vi "kpro 2016.vi"(0 "Output KPRO":path=path "c:/junk.dat", 1 "Initialize":bool, 2 "Finished In":bool, 5 "Absolute Depth In":sgl format="%.2f", 7 "Total Volume In":dbl format="%.2f", 9 "Zeroed Pressure":dbl format="%.2f", 11 "Flow":dbl format="%.2f", 12 "Read String Pot":bool, 13 "Increment":bool, 14 "SS In":i32) -> (4 "Finished Out":bool, 6 "SS Out":i32, 8 "Current Depth Out":sgl format="%.2f", 10 "Total Volume Out":dbl format="%.2f", 15 "Output Array":dbl[][](array[numeric])=[[17182499.0, -1.0, -1.0, 0.07295542423579193, 10.0, 30.0, 1.0, 0.2942041776993234, 33.989999999999995], [17194122.0, -2.0, -2.0, 0.08603630732168976, 10.0, 30.0, 1.0, 0.28579594169762795, 34.989999999999995], [17196835.0, -3.0, -3.0, 0.36859565057132326, 10.0, 30.0, 1.0, 0.27785495971103086, 35.989999999999995], [17198861.0, -4.0, -4.0, 0.493583415597236, 10.0, 30.0, 1.0, 0.27034333603676675, 36.989999999999995], [17203069.0, -5.0, -5.0, 0.23764258555133078, 10.0, 30.0, 1.0, 0.2632271650434325, 37.989999999999995], [17204351.0, -6.0, -6.0, 0.7800312012480499, 10.0, 30.0, 1.0, 0.2564760194921775, 38.989999999999995], [17205734.0, -7.0, -7.0, 0.7230657989877078, 10.0, 30.0, 1.0, 0.25006251562890724, 39.989999999999995], [17206879.0, -8.0, -8.0, 0.8733624454148472, 10.0, 30.0, 1.0, 0.24396194193705784, 40.989999999999995], [17208211.0, -9.0, -9.0, 0.7507507507507507, 10.0, 30.0, 1.0, 0.23815194093831868, 41.989999999999995], [17211804.0, -10.0, -10.0, 0.27831895352073477, 10.0, 30.0, 1.0, 0.23261223540358225, 42.989999999999995], [17214313.0, -11.0, -11.0, 0.3985651654045437, 10.0, 30.0, 1.0, 0.22732439190725168, 43.989999999999995], [17215593.0, -12.0, -12.0, 0.78125, 10.0, 30.0, 1.0, 0.22227161591464772, 44.989999999999995], [17216822.0, -13.0, -13.0, 0.8136696501220504, 10.0, 30.0, 1.0, 0.21743857360295718, 45.989999999999995], [17218103.0, -14.0, -14.0, 0.7806401249024201, 10.0, 30.0, 1.0, 0.2128112364332837, 46.989999999999995], [17219267.0, -15.0, -15.0, 0.859106529209622, 10.0, 30.0, 1.0, 0.20837674515524068, 47.989999999999995], [17220448.0, -16.0, -16.0, 0.8467400508044031, 10.0, 30.0, 1.0, 0.20412329046744235, 48.989999999999995], [17221627.0, -17.0, -17.0, 0.8481764206955046, 10.0, 30.0, 1.0, 0.20004000800160035, 49.989999999999995], [17222775.0, -18.0, -18.0, 0.8710801393728224, 10.0, 30.0, 1.0, 0.19611688566385568, 50.989999999999995], [17223888.0, -19.0, -19.0, 0.8984725965858041, 10.0, 30.0, 1.0, 0.19234468166955185, 51.989999999999995], [17225019.0, -20.0, -20.0, 0.8841732979664014, 10.0, 30.0, 1.0, 0.18871485185884132, 52.989999999999995], [17226151.0, -21.0, -21.0, 0.88339222614841, 10.0, 30.0, 1.0, 0.18521948508983146, 53.989999999999995], [17227282.0, -22.0, -22.0, 0.8841732979664014, 10.0, 30.0, 1.0, 0.18185124568103292, 54.989999999999995]] format="%.5f")   [LabVIEW 2016]
uses:
  Waterloo DAQ/controls/Kpro hydraulic measurement cluster.ctl
  Waterloo DAQ/controls/MCC DAQ Readings.ctl
  KPRO_lv2015/Kpro Globals.vi
  <vilib>/Utility/file.llb/Write Delimited Spreadsheet (DBL).vi
panel:
  in  "String Pot \nSlope":dbl=1.7339999675750732 format="%.2f"
  in  "Sensor Cluster In":T1
  in  "Cluster":T2
  out "Current Absolute Depth":dbl
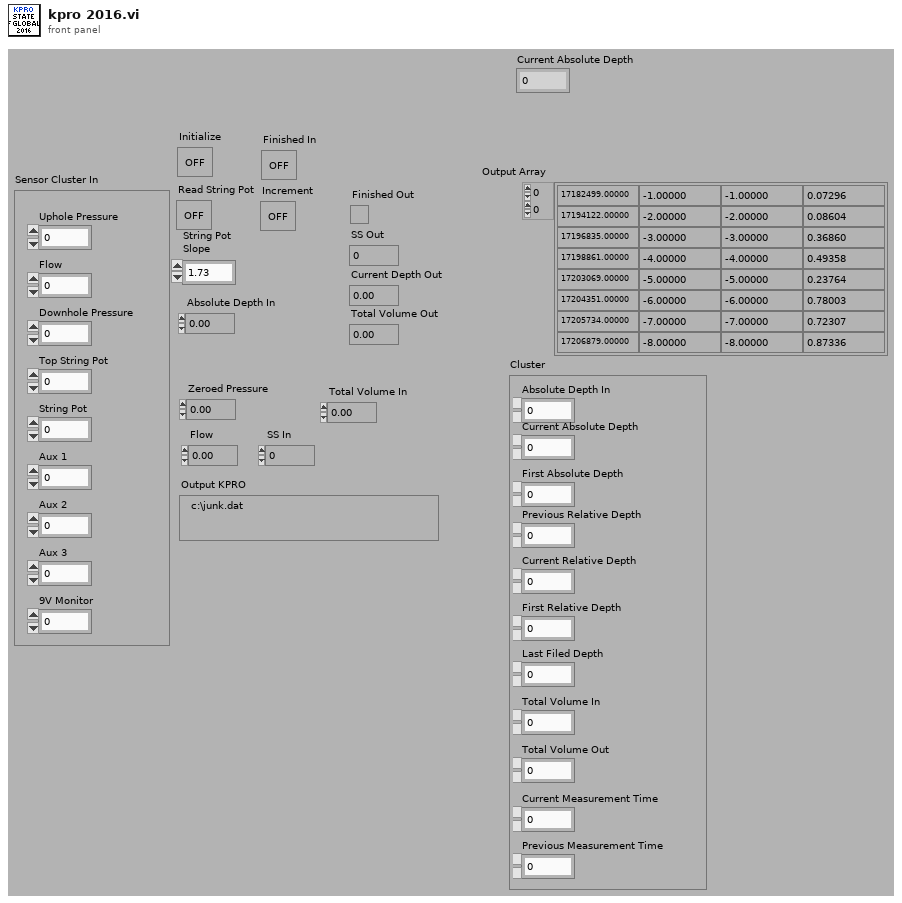
[diagram p1: front panel]
types:
  T1 = typedef "MCC DAQ Readings.ctl" = cluster{"Uphole Pressure":dbl, "Flow":dbl, "Downhole Pressure":dbl, "Top String Pot":dbl, "String Pot":dbl, "Aux 1":dbl, "Aux 2":dbl, "Aux 3":dbl, "9V Monitor":dbl}
  T2 = typedef "Kpro hydraulic measurement cluster.ctl" = cluster{"Absolute Depth In":dbl, "Current Absolute Depth":dbl, "First Absolute Depth":dbl, "Previous Relative Depth":dbl, "Current Relative Depth":dbl, "First Relative Depth":dbl, "Last Filed Depth":dbl, "Total Volume In":dbl, "Total Volume Out":dbl, "Current Measurement Time":dbl, "Previous Measurement Time":dbl}
  T3 = enum16{"Initialize", "Read", "Calc IK and generate Array", "Write Data & finish"}
  T4 = enum16{"Initialize", "Read", "read2", "Write Data & finish"}
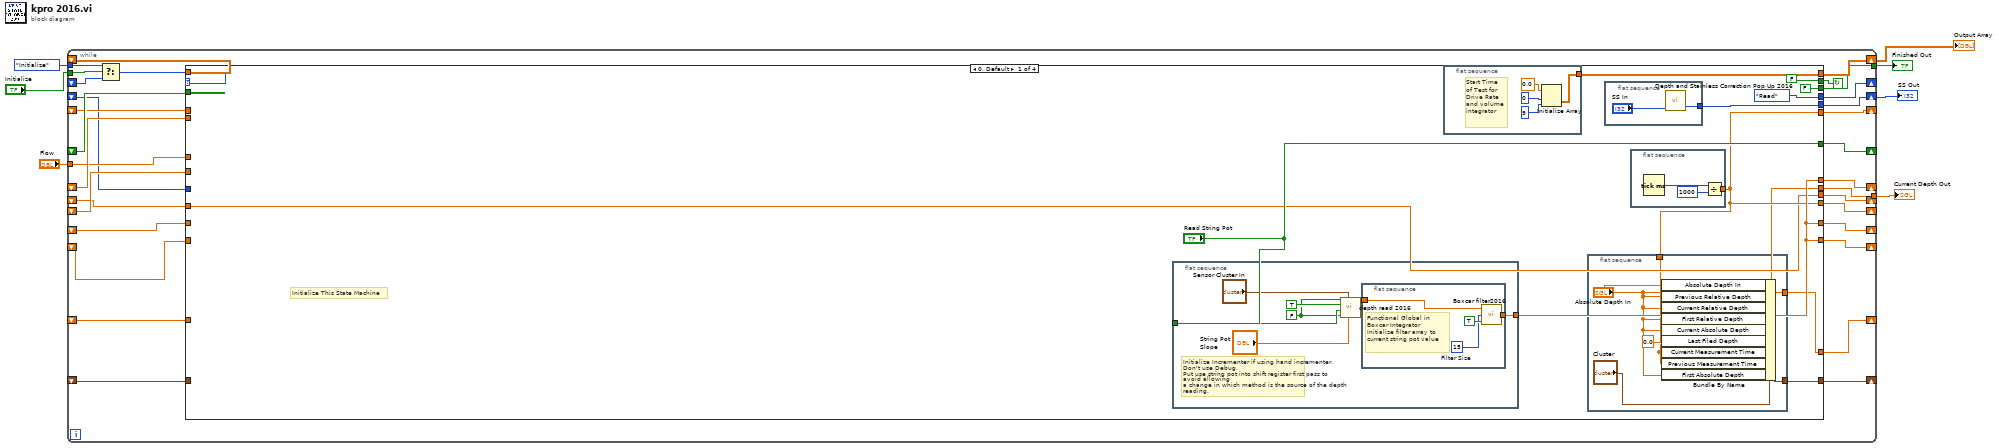
[diagram p0: block diagram]
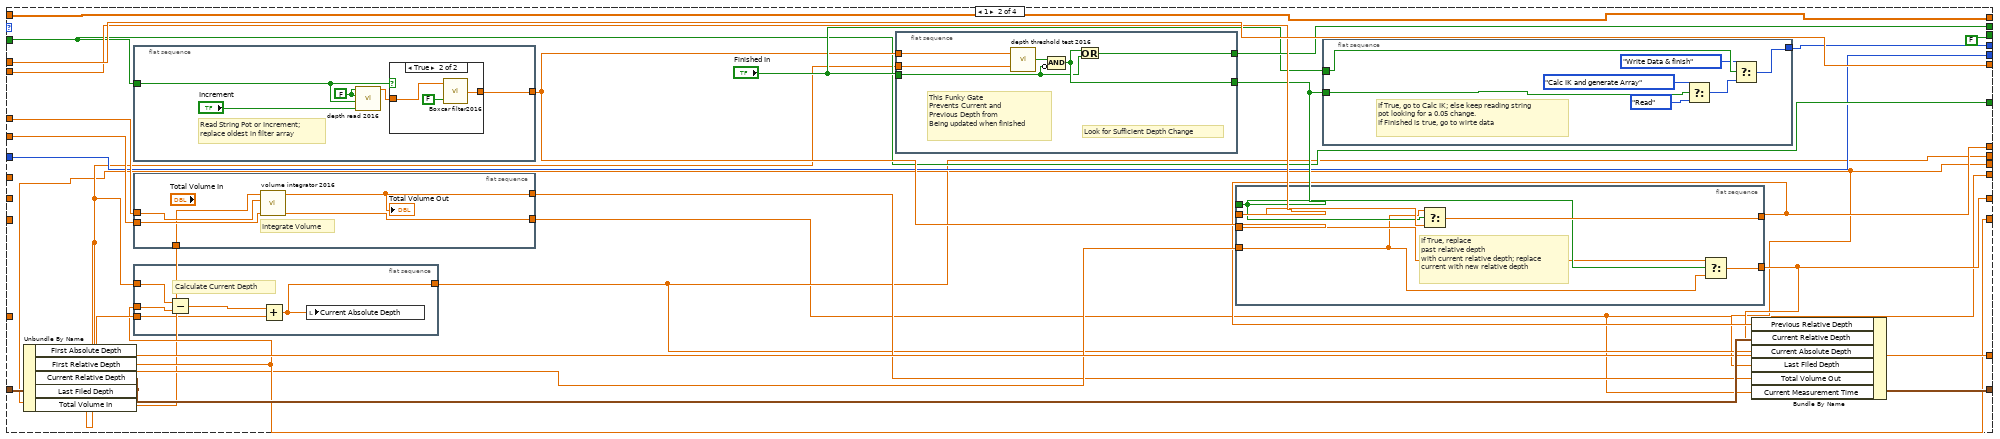
[diagram p2: hidden frame]
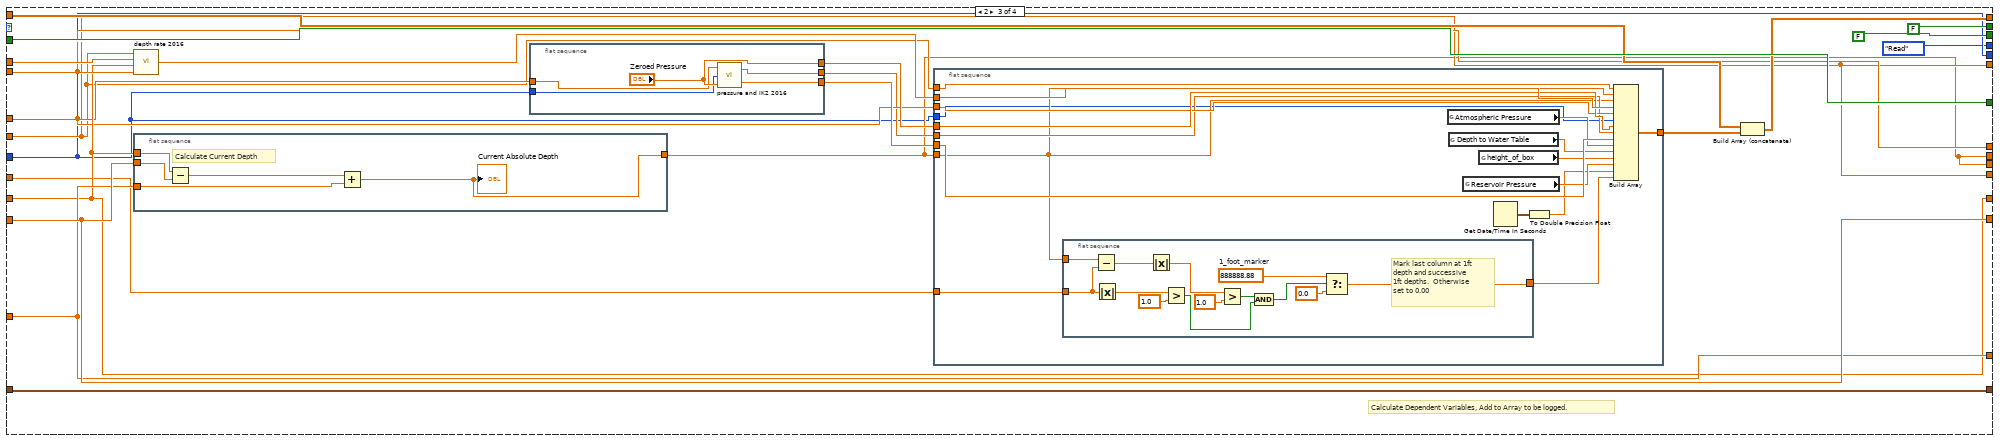
[diagram p4: hidden frame]
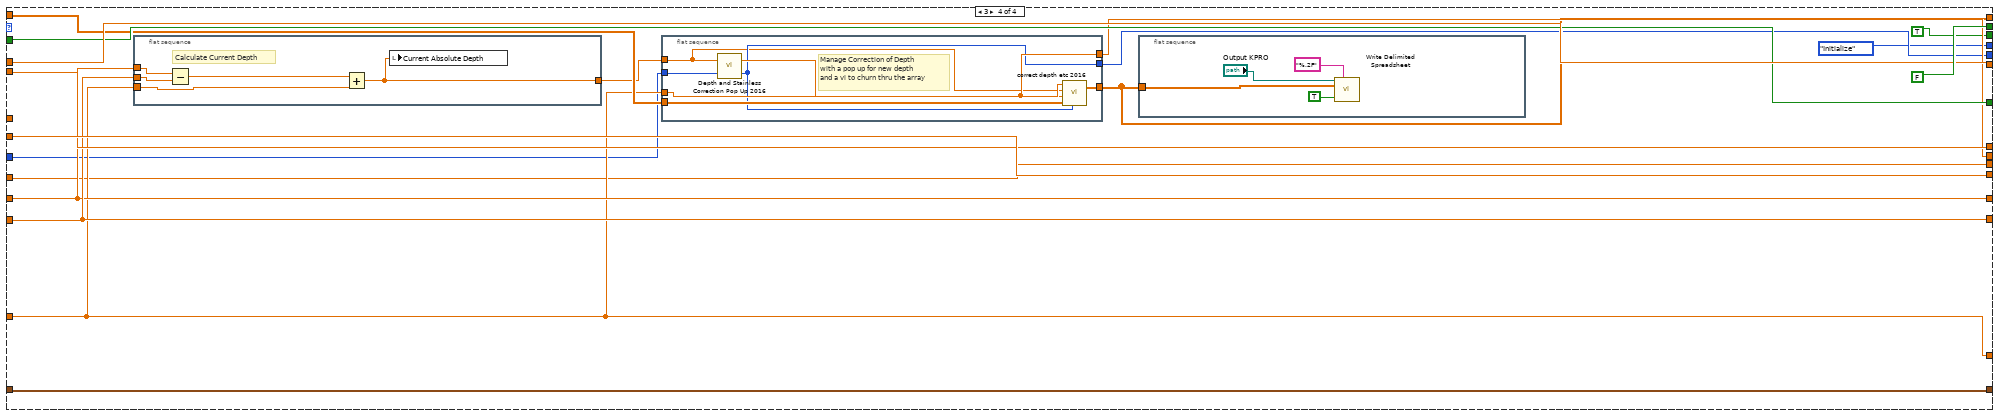
[diagram p5: hidden frame]
diagram:
  n1 = while {
    shift-left: _ -> [w15]
    shift-right: [w16] -> _
    shift-left: _ -> [w18]
    shift-right: [w17] -> w2
    tunnel: [w19] -> w3
    tunnel: [w20] -> w4
    shift-left: _ -> [w21]
    shift-right: [w22] -> _
    shift-left: _ -> [w23]
    shift-right: [w24] -> w1
    shift-left: _ -> [w25]
    shift-right: [w26] -> _
    tunnel: "Flow" -> [w28]
    shift-left: _ -> [w30]
    shift-right: [w31] -> _
    shift-left: _ -> [w29]
    shift-right: [w32] -> _
    shift-left: _ -> [w27]
    shift-right: [w33] -> _
    shift-left: _ -> [w34]
    shift-right: [w35] -> _
    shift-left: _ -> [w36]
    shift-right: [w37] -> _
    tunnel: "Initialize" -> [w38]
    tunnel: T3."Initialize" -> [w13]
    shift-left: _ -> [w11]
    shift-right: [w10] -> _
    shift-right: [w9] -> _
    shift-left: _ -> [w8]
    stop <- w14 continue-if-true
    n2 = Select(t=w13, s=w38, f=w11) -> (s? t:f=w12:u16)
    n3 = case shown="0, Default" w12 {
      tunnel: [T4."Read" w97 T3."Read" T3."Initialize"] -> w10
      tunnel: [w48 w83 w151 w212] -> w37
      tunnel: w36 -> [_ _ w151 w212]
      tunnel: ["Read String Pot" w88 w159 w214] -> w35
      tunnel: w34 -> [_ w88 w159 w214]
      tunnel: [w41 w98 w143 w215] -> w33
      tunnel: [w41 w75 w143 w216] -> w32
      tunnel: [w48 w79 w153 w213] -> w31
      tunnel: w30 -> [_ w94 w153 w213]
      tunnel: w29 -> [_ w96 w143 w216]
      tunnel: w28 -> [_ w95 w145 _]
      tunnel: w27 -> [_ w98 w154 w215]
      tunnel: [w48 w78 w147 w211] -> w26
      tunnel: w25 -> [_ _ w147 w211]
      tunnel: [w47 w99 w156 w207] -> w24
      tunnel: w23 -> [_ w99 w157 w210]
      tunnel: [w39 w84 w150 w208] -> w22
      tunnel: w21 -> [_ _ w150 w208]
      tunnel: [w39 w77 w142 w209] -> w20
      tunnel: [FALSE w93 FALSE FALSE] -> w14
      tunnel: [FALSE FALSE FALSE TRUE] -> w19
      tunnel: w18 -> [_ w87 w140 w205]
      tunnel: [w44 w87 w140 w204] -> w17
      tunnel: [w40 w76 w142 w203] -> w16
      tunnel: w15 -> [w40 _ w141 w203]
      tunnel: [w42 w86 w138 w200] -> w9
      tunnel: w8 -> [_ w85 w138 w200]
      frame 0, Default {
        # "Initialize This State Machine"
        n4 = flat-sequence {
          tunnel: "Read String Pot" -> [w64]
          tunnel: [w62] -> w48
          frame #0 {
            w63 = FALSE
            # "Initialize Incrementer if using hand incrementer,\nDon't use Debug,\nPut use string pot into shift register first pass to avoid allowing\na change in which method is the source of the depth reading."
            n5 = call "depth read 2016.vi"("String Pot \nSlope"="String Pot \nSlope", "Sensor Cluster In"="Sensor Cluster In", "Increment Button"=w63, "Read String Pot"=w64, "Initialize Debug"=TRUE, "Debug"=w63) -> ("Distance"=w66:dbl)  [unwired: 5 in]
            n6 = flat-sequence {
              tunnel: w66 -> [w68]
              tunnel: [w67] -> w62
              frame #0 {
                w69 = 15  # Filter Size
                # "Functional Global in \nBoxcar Integrator\nInitialize filter array to \ncurrent string pot value"
                n7 = call "Boxcar filter2016.vi"("Initialize"=TRUE, "Filter Size"=w69, "Filter Input"=w68) -> ("Filter Output"=w67:dbl)
              }
            }
          }
        }
        n8 = flat-sequence {
          tunnel: [w74] -> w47
          frame #0 {
            # "Start Time\nof Test for\nDrive Rate\nand volume\nintegrator"
            n9 = Initialize Array(0.0, 0, 9) -> (w74:dbl[][])
          }
        }
        n10 = flat-sequence {
          tunnel: [w56] -> w42
          tunnel: w41 -> [w54]
          tunnel: ["Absolute Depth In"] -> w39
          frame #0 {
            n11 = Bundle By Name(cluster="Cluster", "Absolute Depth In"="Absolute Depth In", "Previous Relative Depth"="Absolute Depth In", "Current Relative Depth"="Absolute Depth In", "First Relative Depth"="Absolute Depth In", "Current Absolute Depth"="Absolute Depth In", "Last Filed Depth"=0.0, "Current Measurement Time"=w54, "Previous Measurement Time"=w54, "First Absolute Depth"="Absolute Depth In") -> (w56:T2)
          }
        }
        n12 = flat-sequence {
          tunnel: [w50] -> w44
          frame #0 {
            n13 = call "Depth and Stainless Correction Pop Up 2016.vi"("New Number\n of Stainless\n(Count)"="SS In") -> ("Feet of\nStainless to be\nUsed (Count)"=w50:i32)  [unwired: 1 in, 1 out]
          }
        }
        n14 = flat-sequence {
          tunnel: [w57] -> w41
          frame #0 {
            n15 = Tick Count (ms)() -> (millisecond timer value=w59:u32)
            n16 = Divide(x=w59, y=u32 1000) -> (x/y=w57:dbl)
          }
        }
      }
      frame 1 {
        n17 = Unbundle By Name(w85) -> ("First Absolute Depth"=w84:dbl, "First Relative Depth"=w83:dbl, "Current Relative Depth"=w82:dbl, "Last Filed Depth"=w76:dbl, "Total Volume In"=w81:dbl)
        n18 = flat-sequence {
          tunnel: [w112] -> w89
          tunnel: w88 -> [w111]
          frame #0 {
            w114 = FALSE
            # "Read String Pot or Increment;\nreplace oldest in filter array"
            n19 = call "depth read 2016.vi"("Increment Button"="Increment", "Read String Pot"=w111, "Initialize Debug"=w114, "Debug"=w114) -> ("Distance"=w115:dbl)  [unwired: 7 in]
            n20 = case shown="True" w111 {
              tunnel: w115 -> [w116 w118]
              tunnel: [w116 w117] -> w112
              frame False {
              }
              frame True {
                n21 = call "Boxcar filter2016.vi"("Initialize"=FALSE, "Filter Input"=w118) -> ("Filter Output"=w117:dbl)  [unwired: 1 in]
              }
            }
          }
        }
        n22 = flat-sequence {
          tunnel: w96 -> [w110]
          tunnel: [w109] -> w75
          tunnel: w95 -> [w108]
          tunnel: w81 -> [w107]
          tunnel: [w106] -> w80
          frame #0 {
            # "Integrate Volume"
            n23 = call "volume integrator 2016.vi"("Previous Time (sec)"=w110, "Flow"=w108, "Total Volume in"=w107) -> ("Current Time (sec)"=w109:dbl, "Total Volume Out"=w106:dbl)  [unwired: 3 in]
            "Total Volume Out" <- w106
          }
        }
        n24 = flat-sequence {
          tunnel: w83 -> [w137]
          tunnel: w84 -> [w135]
          tunnel: w82 -> [w134]
          tunnel: [w133] -> w77
          frame #0 {
            # "Calculate Current Depth"
            n25 = Subtract(x=w134, y=w137) -> (x-y=w136:dbl)
            n26 = Add(x=w136, y=w135) -> (x+y=w133:dbl)
            n27 = local write "Current Absolute Depth"(w133) -> ()
          }
        }
        n28 = flat-sequence {
          tunnel: [w124] -> w93
          tunnel: [w123] -> w92
          tunnel: "Finished In" -> [w122]
          tunnel: w89 -> [w121]
          tunnel: w82 -> [w120]
          frame #0 {
            # "Look for Sufficient Depth Change"
            # "This Funky Gate\nPrevents Current and \nPrevious Depth from \nBeing updated when finished"
            n29 = call "depth threshold test 2016.vi"("Depth\nPrevious"=w120, "Depth \nCurrent"=w121) -> ("Threshold\nExceeded"=w125:bool)
            n30 = Compound Arithmetic op=AND(w125, invert w122) -> (w123:bool)
            n31 = Or(x=w123, y=w122) -> (x .or. y?=w124:bool)
          }
        }
        n32 = flat-sequence {
          tunnel: [w105] -> w79
          tunnel: w94 -> [w104]
          tunnel: [w103] -> w78
          tunnel: w92 -> [w102]
          tunnel: w89 -> [w101]
          tunnel: w82 -> [w100]
          frame #0 {
            # "If True, replace\npast relative depth\nwith current relative depth; replace\ncurrent with new relative depth"
            n33 = Select(t=w100, s=w102, f=w104) -> (s? t:f=w105:dbl)
            n34 = Select(t=w101, s=w102, f=w100) -> (s? t:f=w103:dbl)
          }
        }
        n35 = flat-sequence {
          tunnel: [w132] -> w97
          tunnel: w92 -> [w130]
          tunnel: "Finished In" -> [w129]
          frame #0 {
            # "If True, go to Calc IK; else keep reading string pot looking for a 0.05 change.\nIf Finished is true, go to wirte data"
            n36 = Select(t=T3."Calc IK and generate Array", s=w130, f=T3."Read") -> (s? t:f=w131:T3)
            n37 = Select(t=T3."Write Data & finish", s=w129, f=w131) -> (s? t:f=w132:T3)
          }
        }
        n38 = Bundle By Name(cluster=w85, "Previous Relative Depth"=w79, "Current Relative Depth"=w78, "Current Absolute Depth"=w77, "Last Filed Depth"=w76, "Total Volume Out"=w80, "Current Measurement Time"=w75) -> (w86:T2)
      }
      frame 2 {
        # "Calculate Dependent Variables, Add to Array to be logged."
        n39 = call "depth rate 2016.vi"("Depth Last"=w153, "Depth Current"=w147, "Time Last"=w154, "Time Current"=w143) -> ("Depth Rate"=w152:dbl)
        n40 = flat-sequence {
          tunnel: w151 -> [w198]
          tunnel: w150 -> [w197]
          tunnel: w147 -> [w196]
          tunnel: [w195] -> w142
          frame #0 {
            # "Calculate Current Depth"
            n41 = Subtract(x=w196, y=w198) -> (x-y=w199:dbl)
            n42 = Add(x=w199, y=w197) -> (x+y=w195:dbl)
            "Current Absolute Depth" <- w195
          }
        }
        n43 = flat-sequence {
          tunnel: [w194] -> w158
          tunnel: ["Zeroed Pressure"] -> w149
          tunnel: w145 -> [w192]
          tunnel: [w191] -> w144
          tunnel: w140 -> [w190]
          frame #0 {
            n44 = call "pressure and IK2 2016.vi"("Pressure"="Zeroed Pressure", "Ft. of SS"=w190, "flow"=w192) -> ("Corrected Headloss"=w194:dbl, "IK"=w191:dbl)
          }
        }
        n45 = flat-sequence {
          tunnel: w158 -> [w176]
          tunnel: [w175] -> w155
          tunnel: w152 -> [w174]
          tunnel: w149 -> [w173]
          tunnel: w145 -> [w172]
          tunnel: w144 -> [w171]
          tunnel: w143 -> [w166]
          tunnel: w142 -> [w164]
          tunnel: w141 -> [w162]
          tunnel: w140 -> [w160]
          frame #0 {
            n46 = flat-sequence {
              tunnel: w164 -> [w189]
              tunnel: [w183] -> w163
              tunnel: w162 -> [w179]
              frame #0 {
                w185 = 888888.88  # 1_foot_marker
                # "Mark last column at 1ft \ndepth and successive\n1ft depths.  Otherwise\nset to 0.00"
                n47 = Subtract(x=w189, y=w179) -> (x-y=w188:dbl)
                n48 = Absolute Value(x=w179) -> (abs(x)=w177:dbl)
                n49 = Absolute Value(x=w188) -> (abs(x)=w186:dbl)
                n50 = Greater?(x=w177, y=1.0) -> (0:w180:bool)
                n51 = Greater?(x=w186, y=1.0) -> (0:w181:bool)
                n52 = And(x=w181, y=w180) -> (x .and. y?=w182:bool)
                n53 = Select(t=w185, s=w182, f=0.0) -> (s? t:f=w183:dbl)
              }
            }
            n54 = global read "Kpro Globals.vi" "Atmospheric Pressure"() -> (w170:dbl)
            n55 = global read "Kpro Globals.vi" "Depth to Water Table"() -> (w168:dbl)
            n56 = global read "Kpro Globals.vi" "Reservoir Pressure"() -> (w169:dbl)
            n57 = global read "Kpro Globals.vi" "height_of_box"() -> (w167:dbl)
            n58 = Get Date/Time In Seconds() -> (seconds since 1Jan1904=w161:timestamp)
            n59 = To Double Precision Float(number=w161) -> (double precision float=w165:dbl)
            n60 = Build Array(w166, w164, w164, w174, w172, w160, w173, w171, w176, w170, w168, w167, w169, w165, w163) -> (w175:dbl[])
          }
        }
        n61 = Build Array (concatenate)(w157, w155) -> (w156:dbl[][])
      }
      frame 3 {
        n62 = flat-sequence {
          tunnel: w212 -> [w228]
          tunnel: w211 -> [w227]
          tunnel: w208 -> [w226]
          tunnel: [w225] -> w202
          frame #0 {
            # "Calculate Current Depth"
            n63 = Subtract(x=w227, y=w228) -> (x-y=w229:dbl)
            n64 = Add(x=w229, y=w226) -> (x+y=w225:dbl)
            n65 = local write "Current Absolute Depth"(w225) -> ()
          }
        }
        n66 = flat-sequence {
          tunnel: w210 -> [w224]
          tunnel: [w223] -> w209
          tunnel: w208 -> [w222]
          tunnel: [w221] -> w207
          tunnel: w205 -> [w220]
          tunnel: [w219] -> w204
          tunnel: w202 -> [w218]
          frame #0 {
            # "Manage Correction of Depth\nwith a pop up for new depth\nand a vi to churn thru the array"
            n67 = call "Depth and Stainless Correction Pop Up 2016.vi"("New Number\n of Stainless\n(Count)"=w220, "Input \nCorrected \nDepth (Feet)"=w218) -> ("Feet of\nStainless to be\nUsed (Count)"=w219:i32, "Depth to \nbe Used \n(Feet)"=w223:sgl)
            n68 = call "correct depth etc 2016.vi"("Correct Depth"=w223, "Incorrect Depth"=w218, "First Absolute Depth"=w222, "Uncorrected Array"=w224, "New Stainless Feet"=w219) -> ("Corrected Array"=w221:dbl[][])  [unwired: 1 in]
          }
        }
        n69 = flat-sequence {
          tunnel: w207 -> [w232]
          frame #0 {
            n70 = call-poly <vilib>:"Write Delimited Spreadsheet.vi"("file path (dialog if empty)"="Output KPRO", "format (%.3f)"="%.2F", "2D data"=w232, "append to file? (new file:F)"=TRUE) -> ()  [unwired: 10 in, 2 out]
          }
        }
      }
    }
  }
  "Current Depth Out" <- w4
  "Finished Out" <- w3
  "SS Out" <- w2
  "Output Array" <- w1
